vi "Determine Warning Case Structures.vi"() -> ()   [LabVIEW 2014]
panel:
  out "Warning?":bool
  out "Warning Text":string
  in  "Min Temp":dbl
  in  "Max Temp":dbl
  in  "Current Temp":dbl
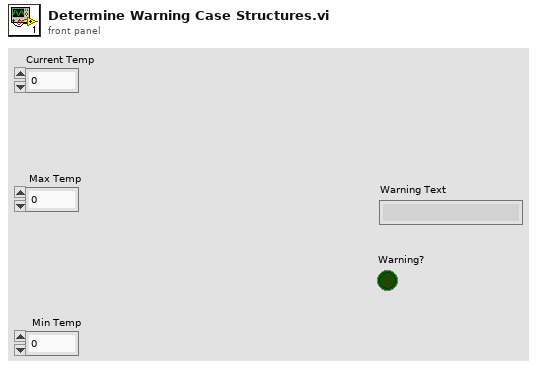
[diagram p1: front panel]
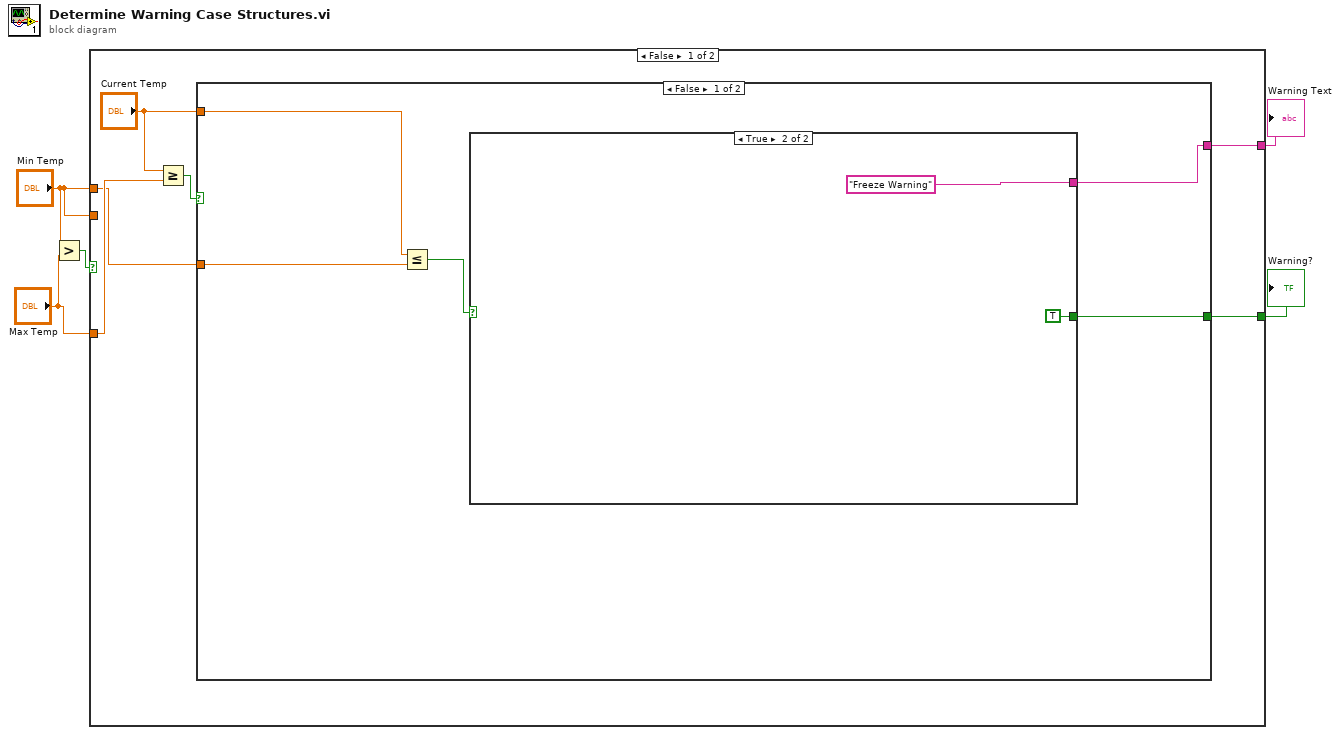
[diagram p0: block diagram]
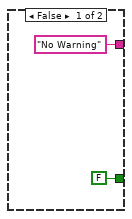
[diagram p2: hidden frame]
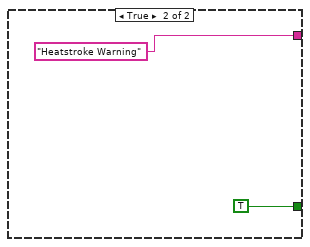
[diagram p3: hidden frame]
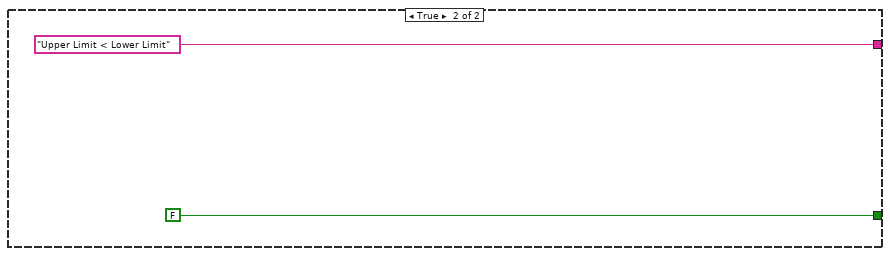
[diagram p4: hidden frame]
diagram:
  n1 = Greater?(x="Min Temp", y="Max Temp") -> (0:w2:bool)
  n2 = case shown="False" w2 {
    tunnel: "Max Temp" -> [w10 _]
    tunnel: "Min Temp" -> [_ _]
    tunnel: [w9 "Upper Limit < Lower Limit"] -> w5
    tunnel: [w6 FALSE] -> w4
    tunnel: "Min Temp" -> [w7 _]
    frame False {
      n3 = Greater Or Equal?(x="Current Temp", y=w10) -> (x >= y?=w11:bool)
      n4 = case shown="False" w11 {
        tunnel: [w13 "Heatstroke Warning"] -> w9
        tunnel: "Current Temp" -> [w16 _]
        tunnel: w7 -> [w15 _]
        tunnel: [w12 TRUE] -> w6
        frame False {
          n5 = Less Or Equal?(x=w16, y=w15) -> (x <= y?=w14:bool)
          n6 = case shown="True" w14 {
            tunnel: ["No Warning" "Freeze Warning"] -> w13
            tunnel: [FALSE TRUE] -> w12
            frame False {
            }
            frame True {
            }
          }
        }
        frame True {
        }
      }
    }
    frame True {
    }
  }
  "Warning Text" <- w5
  "Warning?" <- w4
